vi "Periodic Tasks.vi"(8 "error in":errorcluster) -> ()   [LabVIEW 2015]
doc: "This VI runs in parallel to other tasks. It can contain as many user-defined periodic loops as you need. These can carry out PID or other sorts of timed response."
uses:
  <vilib>/Rock Robotics/WPI/Utilities/WPI_GetSetVariantRefNum.vi
  Robot Global Data.vi
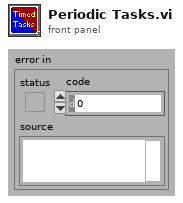
[diagram p1: front panel]
types:
  T1 = typedef "WPI_SwitchDevRef.ctl" = cluster{"DevStatus":errorcluster, "DIO Channel":T2, "CntIndex":T3, "Normally Closed":bool}
  T2 = typedef "FPGA_DIOChannel.ctl" = enum8{"DIO 0", "DIO 1", "DIO 2", "DIO 3", "DIO 4", "DIO 5", "DIO 6", "DIO 7", "DIO 8", "DIO 9", "DIO MXP 0", "DIO MXP 1", "DIO MXP 2", "DIO MXP 3", "DIO MXP 4", "DIO MXP 5", "DIO MXP 6", "DIO MXP 7", "DIO MXP 8", "DIO MXP 9", "DIO MXP 10", "DIO MXP 11", "DIO MXP 12", "DIO MXP 13", "DIO MXP 14", "DIO MXP 15", "Invalid"}
  T3 = typedef "FPGA_CounterCtrSystemIndex.ctl" = enum8{"Ctr 0", "Ctr 1", "Ctr 2", "Ctr 3", "Ctr 4", "Ctr 5", "Ctr 6", "Ctr 7", "Invalid"}
  T4 = typedef "WPI_ServoDeviceRef.ctl" = cluster{"DeviceStatus":errorcluster, "PWM Channel":T5, "DeadBand":T6}
  T5 = typedef "FPGA_DIOPWMChannel.ctl" = enum8{"PWM 0", "PWM 1", "PWM 2", "PWM 3", "PWM 4", "PWM 5", "PWM 6", "PWM 7", "PWM 8", "PWM 9", "PWM MXP 0", "PWM MXP 1", "PWM MXP 2", "PWM MXP 3", "PWM MXP 4", "PWM MXP 5", "PWM MXP 6", "PWM MXP 7", "PWM MXP 8", "PWM MXP 9", "Invalid"}
  T6 = typedef "WPI_PWMDeadband.ctl" = cluster{"Name":string, "maxPositivePwm":i32, "minPositivePwm":i32, "centerPwm":i32, "maxNegativePwm":i32, "minNegativePwm":i32, "angularRange":u16}
  T7 = typedef "WPI_JoystickDevRef.ctl" = cluster{"Device":T8}
  T8 = typedef "WPI_JoystickDeviceEnum.ctl" = enum16{"USB 0", "USB 1", "USB 2", "USB 3", "USB 4", "USB 5"}
  T9 = cluster{"Buttons[0]":bool, "Buttons[1]":bool, "Buttons[2]":bool, "Buttons[3]":bool, "Buttons[4]":bool, "Buttons[5]":bool, "Buttons[6]":bool, "Buttons[7]":bool, "Buttons[8]":bool}
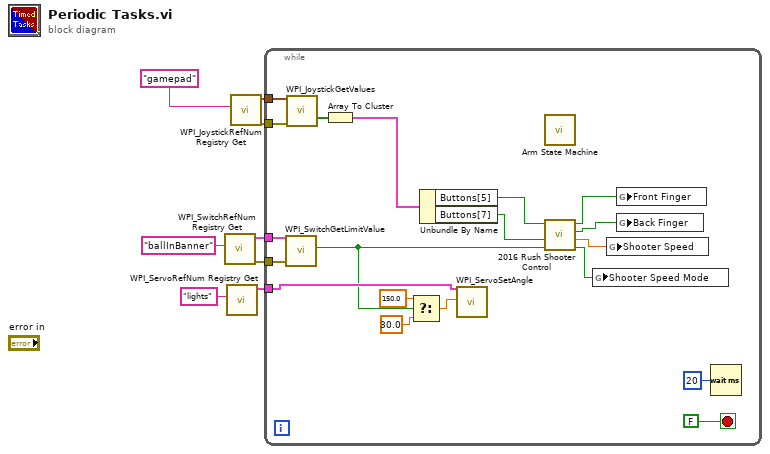
[diagram p0: block diagram]
diagram:
  n1 = call <vilib>:"WPI_SwitchRefNum Registry Get.vi"("refnum name"="ballInBanner") -> ("error out"=w5:errorcluster, "SwitchDevRef"=w6:T1)  [unwired: 9 in]
  n2 = call <vilib>:"WPI_ServoRefNum Registry Get.vi"("refnum name"="lights") -> ("ServoDeviceRef"=w2:T4)  [unwired: 9 in, 1 out]
  n3 = call <vilib>:"WPI_JoystickRefNum Registry Get.vi"("refnum name"="gamepad") -> ("error out"=w3:errorcluster, "JoystickDevRef"=w4:T7)  [unwired: 1 in, 8 out]
  n4 = while {
    tunnel: w6 -> [w22]
    tunnel: w5 -> [w21]
    tunnel: w4 -> [w18]
    tunnel: w3 -> [w17]
    tunnel: w2 -> [w13]
    stop <- FALSE stop-if-true
    n5 = call <vilib>:"WPI_SwitchGetLimitValue.vi"("error in (no error)"=w21, "SwitchDevRef"=w22) -> ("Switch Pressed"=w9:bool)  [unwired: 7 in, 2 out]
    n6 = call <vilib>:"WPI_JoystickGetValues.vi"("error in (no error)"=w17, "JoystickDevRef"=w18) -> ("Buttons"=w19:bool[])  [unwired: 5 in, 4 out]
    n7 = Array To Cluster(array=w19) -> (cluster=w20:T9)
    n8 = Select(t=150.0, s=w9, f=30.0) -> (s? t:f=w12:dbl)
    n9 = Unbundle By Name(w20) -> ("Buttons[5]"=w14:bool, "Buttons[7]"=w16:bool)
    n10 = call <vilib>:"WPI_ServoSetAngle.vi"("Angle"=w12, "ServoDeviceRef"=w13) -> ()  [unwired: 8 in, 2 out]
    n11 = call "Arm State Machine.vi"() -> ()  [unwired: 12 in]
    n12 = call "2016 Rush Shooter Control.vi"("ballInBanner"=w9, "Spin up wheels button"=w16, "Shoot button"=w14) -> ("Shooter Wheel Speed Mode?"=w15:bool, "Shooter wheel speeds"=w25:dbl, "Harvester actuator back"=w23:bool, "Harvester actuator front"=w24:bool)  [unwired: 5 in]
    n13 = global write "Robot Global Data.vi" "Shooter Speed Mode"(w15) -> ()
    n14 = global write "Robot Global Data.vi" "Shooter Speed"(w25) -> ()
    n15 = global write "Robot Global Data.vi" "Front Finger"(w24) -> ()
    n16 = global write "Robot Global Data.vi" "Back Finger"(w23) -> ()
    n17 = Wait (ms)(milliseconds to wait=u32 20) -> ()  [unwired: 1 out]
  }
